vi "Close Gates.vi"(8 "error in (no error)":errorcluster, 11 "gate":T1) -> (0 "error out":errorcluster, 3 "gate out":T1)   [LabVIEW 2015, in "Gates.lvlib"]
doc: "Closes referenced gate."
uses:
  Gates.lvlib
  Gate.ctl
  Gate Pass.ctl
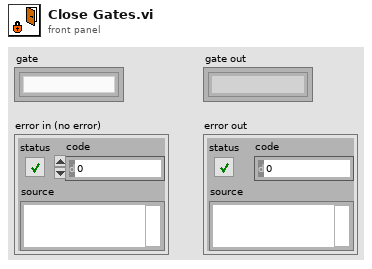
[diagram p1: front panel]
types:
  T1 = typedef "Gates.lvlib/Gate.ctl" = refnum<k1>
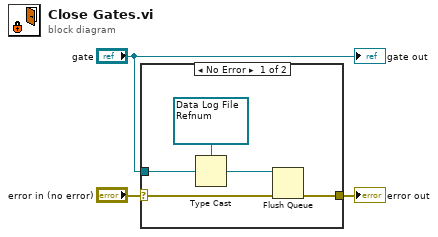
[diagram p0: block diagram]
diagram:
  n1 = case shown="No Error" "error in (no error)" {
    selector: "error in (no error)" -> [w7 w9]
    tunnel: "gate" -> [w8 _]
    tunnel: [w6 w9] -> w1
    frame No Error {
      w5 = refnum<queue> refnum items=["Gate Pass"] ("queue out")
      n2 = Type Cast(type=w5, x=w8) -> (*(type *) &x=w4:refnum<queue>)
      n3 = Flush Queue(queue=w4, error in (no error)=w7) -> (error out=w6:errorcluster)  [unwired: 2 out]
    }
    frame Error {
    }
  }
  "error out" <- w1
  "gate out" <- "gate"
